vi "DataGenerator.vi"() -> (0 "error out":errorcluster)   [LabVIEW 2013]
uses:
  Globals.vi
  <vilib>/gmath/statdist.llb/Normal Random.vi
  <vilib>/gmath/NI_Gmath.lvlib
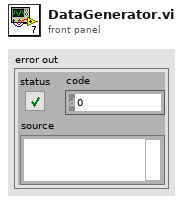
[diagram p1: front panel]
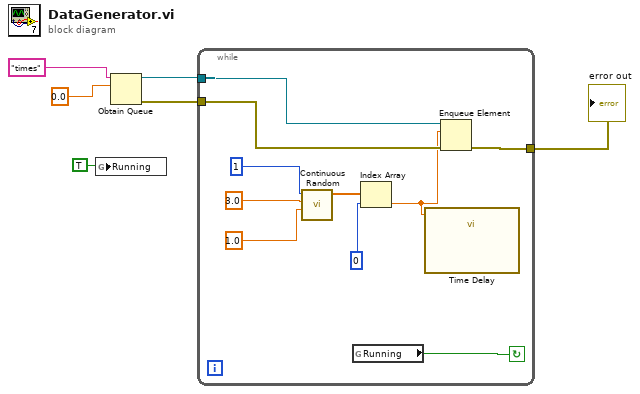
[diagram p0: block diagram]
diagram:
  n1 = global write "Globals.vi" "Running"(TRUE) -> ()
  n2 = Obtain Queue(name (unnamed)="times", element data type=0.0) -> (queue out=w6:refnum<queue>, error out=w4:errorcluster)  [unwired: 3 in, 1 out]
  n3 = while {
    tunnel: w6 -> [w16]
    tunnel: w4 -> [w15]
    tunnel: [w14] -> w3
    stop <- w13 continue-if-true
    n4 = call-poly <vilib>:"Continuous Random.vi"("std"=1.0, "mean"=3.0, "samples"=1) -> ("normal random data"=w9:dbl[])  [unwired: 7 in, 1 out]
    n5 = global read "Globals.vi" "Running"() -> (w13:bool)
    n6 = Index Array(array=w9, index=0) -> (element=w7:dbl)
    n7 = call "Time Delay"("Delay Time (s)"=w7) -> ()  [unwired: 10 in, 1 out]
    n8 = Enqueue Element(queue=w16, element=w7, error in (no error)=w15) -> (error out=w14:errorcluster)  [unwired: 1 in, 2 out]
  }
  "error out" <- w3
